vi "pobiez wart enkodera FVG.vi"(7 "Akcja (Pobrano)":enum16{"Pobierz", "Pobrano", "Czekaj"}(ring)=enum."Pobrano", 8 "error in (no error)":errorcluster, 10 "Impulsy In":dbl) -> (0 "error out":errorcluster, 1 "Flaga":bool, 2 "Impulsy Out":dbl)   [LabVIEW 2013]
doc: "Zmienna funkcjonalna do pobierania aktualnej wartoœci enkodera\ndo pêtli GUI celem obliczenia skali"
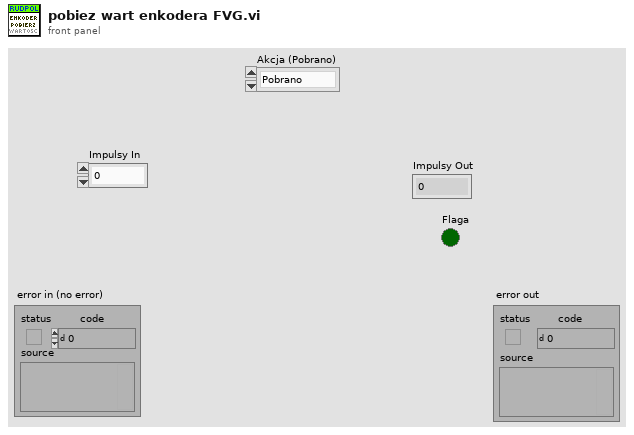
[diagram p1: front panel]
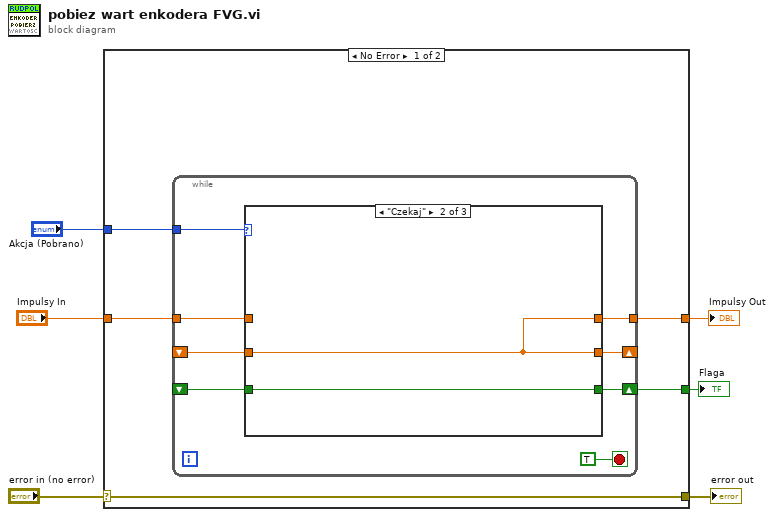
[diagram p0: block diagram]
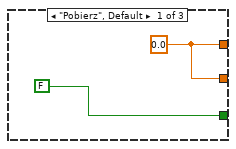
[diagram p2: hidden frame]
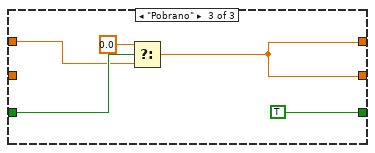
[diagram p3: hidden frame]
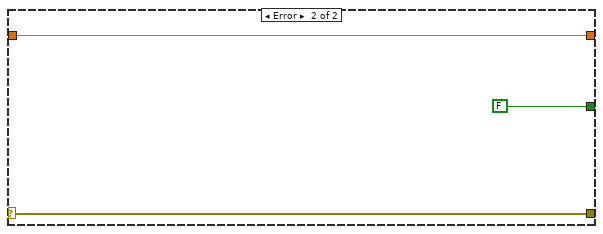
[diagram p4: hidden frame]
diagram:
  n1 = case shown="No Error" "error in (no error)" {
    selector: "error in (no error)" -> [w11 w31]
    tunnel: [w11 w31] -> w5
    tunnel: "Akcja (Pobrano)" -> [w10 _]
    tunnel: "Impulsy In" -> [w9 w30]
    tunnel: [w8 w30] -> w2
    tunnel: [w7 FALSE] -> w1
    frame No Error {
      n2 = while {
        tunnel: w10 -> [w18]
        tunnel: w9 -> [w17]
        shift-right: [w16] -> w7
        shift-left: _ -> [w12]
        tunnel: [w15] -> w8
        shift-right: [w14] -> _
        shift-left: _ -> [w13]
        stop <- TRUE stop-if-true
        n3 = case shown="\"Czekaj\"" w18 {
          tunnel: w17 -> [_ _ w26]
          tunnel: [FALSE w23 TRUE] -> w16
          tunnel: [w20 w22 w25] -> w15
          tunnel: [w20 w22 w25] -> w14
          tunnel: w13 -> [_ w22 _]
          tunnel: w12 -> [_ w23 w27]
          frame "Pobierz", Default {
            w20 = 0.0 ("Impulsy In")
          }
          frame "Czekaj" {
          }
          frame "Pobrano" {
            n4 = Select(t=0.0, s=w27, f=w26) -> (s? t:f=w25:dbl)
          }
        }
      }
    }
    frame Error {
    }
  }
  "error out" <- w5
  "Impulsy Out" <- w2
  "Flaga" <- w1
